vi "to string.vi"(8 "error in":errorcluster, 11 "fixed channel configuration in":refnum<class "WaveformAcq configuration.lvclass">) -> (0 "error out":errorcluster, 1 "data":string, 2 "version":string, 3 "fixed channel configuration out":refnum<class "WaveformAcq configuration.lvclass">)   [LabVIEW 2017, in "WaveformAcq configuration.lvclass"]
doc: "Provides an interface for saving a module configuration to a file or other serialized data source. It is recommended that all children of this class store data in two sets--data required for its own initialization, and any data required for parent initialization--and that each implementation uses the <b>Call Parent Method</b> primitive to serialize parent information.\nNI Tag Bus Module Framework 1.0.3.43\nNI Systems Engineering"
uses:
  WaveformAcq configuration.lvclass
  WaveformAcq configuration.lvclass/WaveformAcq configuration.ctl
  <vilib>/NI/DCAF/Tag Editor Core/control module/configuration/control module configuration.lvclass
  <vilib>/NI/Configuration Framework/serializable configuration/NISE_CEF_serializable configuration.lvclass
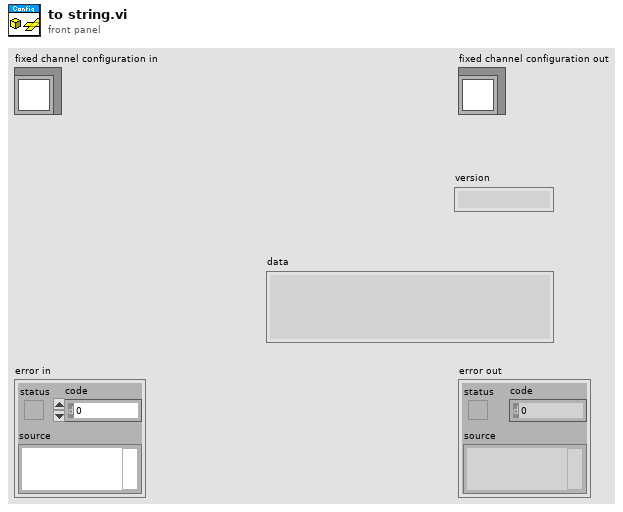
[diagram p1: front panel]
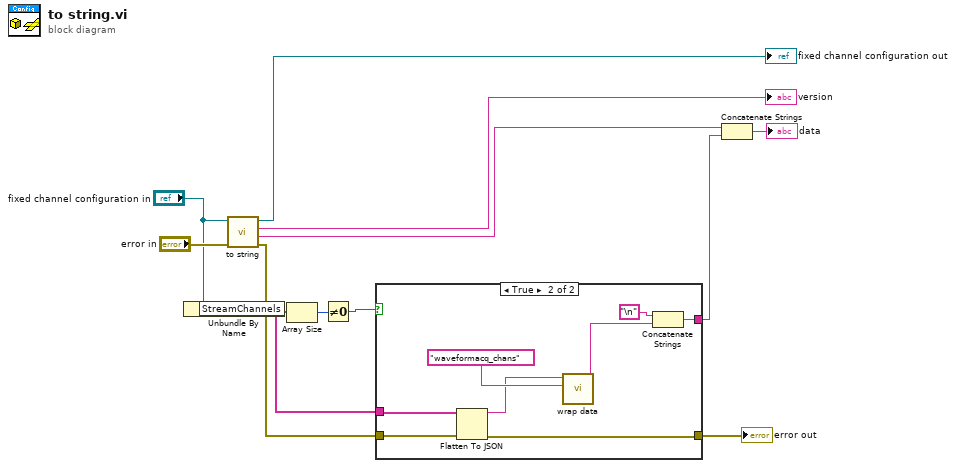
[diagram p0: block diagram]
diagram:
  n1 = Unbundle By Name("fixed channel configuration in") -> ("StreamChannels"=w5:string[])
  n2 = call-parent "to string.vi"("error in"="error in", "fixed channel configuration in"="fixed channel configuration in") -> ("error out"=w9:errorcluster, "data"=w2:string, "version"=→"version":string, "fixed channel configuration out"=→"fixed channel configuration out":refnum<class "WaveformAcq configuration.lvclass">)  [unwired: 6 in]
  n3 = Array Size(array=w5) -> (size(s)=w7:i32)
  n4 = Not Equal To 0?(x=w7) -> (x != 0?=w6:bool)
  n5 = case shown="True" w6 {
    tunnel: [_ w19] -> w1
    tunnel: w5 -> [_ w17]
    tunnel: w9 -> [w13 w16]
    tunnel: [w13 w14] -> w4
    frame False {
    }
    frame True {
      n6 = Flatten To JSON(anything=w17, error in (no error)=w16) -> (JSON string=w15:string, 11:w14:errorcluster)  [unwired: 1 in]
      n7 = call <vilib>:"wrap data.vi"("identifier"="waveformacq_chans", "data to wrap"=w15) -> ("wrapped data"=w20:string)  [unwired: 9 in]
      n8 = Concatenate Strings("\n", w20) -> (w19:string)
    }
  }
  "error out" <- w4
  n9 = Concatenate Strings(w2, w1) -> (→"data":string)
